vi "Handle Ctl[] Settings.vi"(7 "Write Ctl? (F:Read)":bool, 8 "error in (no error)":errorcluster, 10 "Controls[]":refnum<vi>[](array[refnum]), 11 "Save Restore Settings in":refnum<class "Save Restore Settings.lvclass">) -> (0 "error out":errorcluster, 3 "Save Restore Settings out":refnum<class "Save Restore Settings.lvclass">)   [LabVIEW 2020, in "Save Restore Settings.lvclass"]
uses:
  <userlib>/_MGI/Application Control/MGI Save Restore Settings/Save Restore Settings.lvclass
  <userlib>/_MGI/Application Control/MGI Save Restore Settings/Control Info.ctl
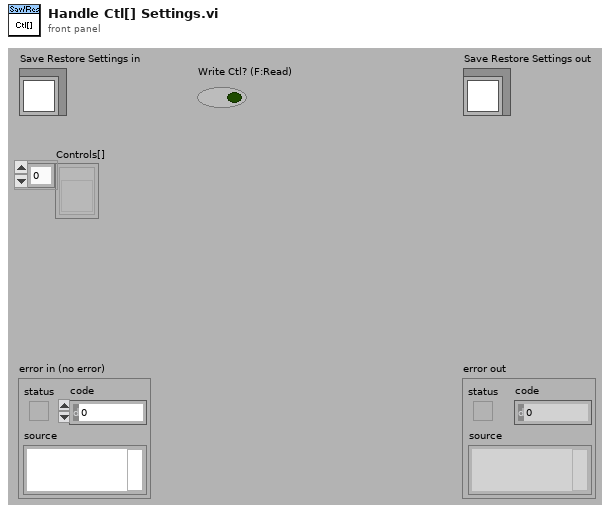
[diagram p1: front panel]
types:
  T1 = typedef "Save Restore Settings.lvclass/Control Info.ctl" = cluster{"Ref":refnum<vi>, "Tag":string}
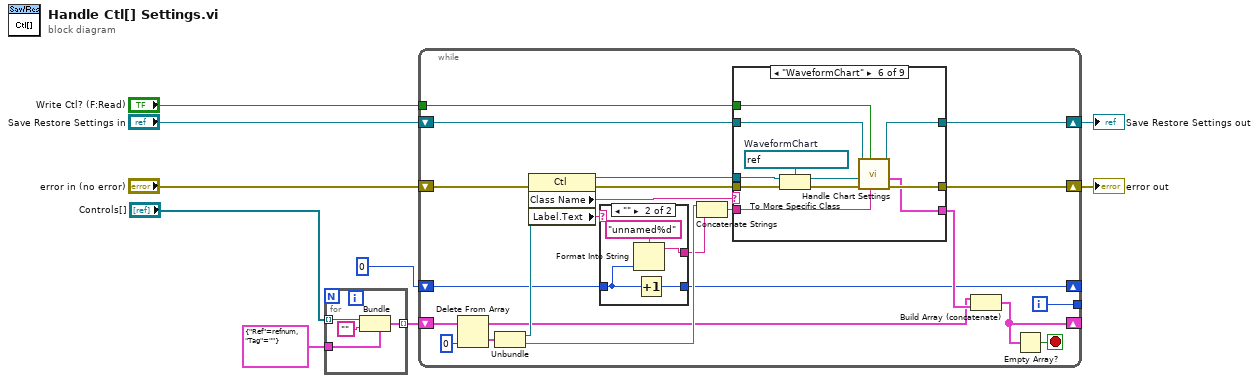
[diagram p0: block diagram]
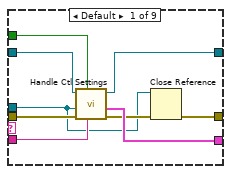
[diagram p3: hidden frame]
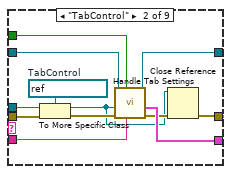
[diagram p4: hidden frame]
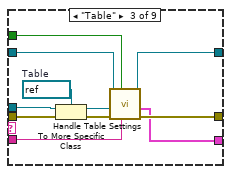
[diagram p5: hidden frame]
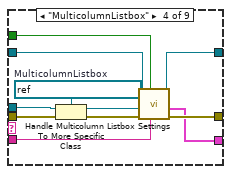
[diagram p6: hidden frame]
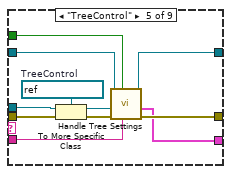
[diagram p7: hidden frame]
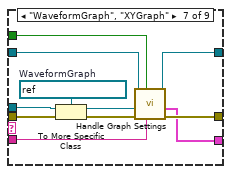
[diagram p8: hidden frame]
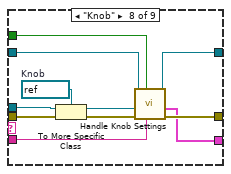
[diagram p9: hidden frame]
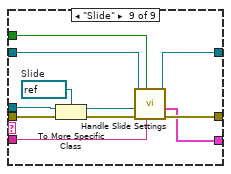
[diagram p10: hidden frame]
diagram:
  n1 = for {
    tunnel: "Controls[]" -> [w13] mode=indexing
    tunnel: [w12] -> w9 mode=indexing
    tunnel: T1 {"Ref"=refnum, "Tag"=""} ("Save Restore Settings.lvclass:Control Info") -> [w10]
    n2 = Bundle(cluster=w10, "Ref"=w13, "Tag"="") -> (w12:T1)
  }
  n3 = while {
    shift-right: [w23] -> _
    shift-left: w9 -> [w36]
    shift-right: [w28] -> w6
    shift-left: "error in (no error)" -> [w29]
    shift-right: [w25] -> w5
    shift-left: "Save Restore Settings in" -> [w26]
    shift-right: [w16] -> _
    shift-left: 0 -> [w18]
    tunnel: [w15] -> _
    tunnel: "Write Ctl? (F:Read)" -> [w14]
    i -> [w15]
    stop <- w27 stop-if-true
    n4 = Delete From Array(array=w36, index=0) -> (deleted portion=w35:T1, array with subset deleted=w20:T1[])  [unwired: 1 in]
    n5 = Unbundle(w35) -> ("Ref"=w22:refnum<vi>, "Tag"=w21:string)
    n6 = property class="Ctl"(reference=w22, error in=w29) -> (reference out=w33:refnum<vi>, error out=w34:errorcluster, "Class Name"=w32:string, "Label.Text"=w19:string)
    n7 = case shown="\"\"" w19 {
      selector: w19 -> [w38 _]
      tunnel: w18 -> [w37 w41]
      tunnel: [w38 w40] -> w17
      tunnel: [w37 w42] -> w16
      frame Default {
      }
      frame "" {
        n8 = Format Into String(format string="unnamed%d", w41) -> (resulting string=w40:string)  [unwired: 2 in, 1 out]
        n9 = Increment(x=w41) -> (x+1=w42:i32)
      }
    }
    n10 = Concatenate Strings(w21, w17) -> (w31:string)
    n11 = case shown="\"WaveformChart\"" w32 {
      tunnel: w34 -> [w51 w63 w73 w84 w95 w106 w117 w128 w139]
      tunnel: w31 -> [w50 w55 w69 w76 w87 w98 w109 w120 w131]
      tunnel: w33 -> [w44 w62 w72 w83 w94 w105 w116 w127 w138]
      tunnel: [w45 w60 w66 w78 w89 w100 w111 w122 w133] -> w28
      tunnel: w26 -> [w49 w59 w68 w81 w92 w103 w114 w125 w136]
      tunnel: [w48 w54 w67 w80 w91 w102 w113 w124 w135] -> w25
      tunnel: [w47 w57 w65 w77 w88 w99 w110 w121 w132] -> w24
      tunnel: w14 -> [w43 w52 w64 w75 w86 w97 w108 w119 w130]
      frame Default {
        n12 = call-dynamic "Handle Ctl Settings.vi"("Control Setting Tag"=w50, "Write? (F:Read)"=w43, "error in (no error)"=w51, "Control"=w44, "Save Restore Settings in"=w49) -> ("error out"=w46:errorcluster, "Sub Controls"=w47:T1[], "Save Restore Settings out"=w48:refnum<class "Save Restore Settings.lvclass">)  [unwired: 4 in]
        n13 = Close Reference(reference=w44, error in (no error)=w46) -> (error out=w45:errorcluster)
      }
      frame "TabControl" {
        w61 = refnum<vi> refnum  # TabControl
        n14 = To More Specific Class(target class=w61, reference=w62, error in=w63) -> (specific class reference=w53:refnum<vi>, error out=w58:errorcluster)
        n15 = call-dynamic "Handle Tab Settings.vi"("Tab Setting Name in"=w55, "Write? (F:Read)"=w52, "error in (no error)"=w58, "Tab"=w53, "Save Restore Settings in"=w59) -> ("error out"=w56:errorcluster, "Sub Controls"=w57:T1[], "Save Restore Settings out"=w54:refnum<class "Save Restore Settings.lvclass">)  [unwired: 4 in]
        n16 = Close Reference(reference=w53, error in (no error)=w56) -> (error out=w60:errorcluster)
      }
      frame "Table" {
        w74 = refnum<vi> refnum  # Table
        n17 = To More Specific Class(target class=w74, reference=w72, error in=w73) -> (specific class reference=w71:refnum<vi>, error out=w70:errorcluster)
        n18 = call-dynamic "Handle Table Settings.vi"("Table Setting Name in"=w69, "Write? (F:Read)"=w64, "error in (no error)"=w70, "Table Ref"=w71, "Save Restore Settings in"=w68) -> ("error out"=w66:errorcluster, "Sub Controls"=w65:T1[], "Save Restore Settings out"=w67:refnum<class "Save Restore Settings.lvclass">)  [unwired: 4 in]
      }
      frame "MulticolumnListbox" {
        w85 = refnum<vi> refnum  # MulticolumnListbox
        n19 = To More Specific Class(target class=w85, reference=w83, error in=w84) -> (specific class reference=w82:refnum<vi>, error out=w79:errorcluster)
        n20 = call-dynamic "Handle Multicolumn Listbox Settings.vi"("Table Setting Name in"=w76, "Write? (F:Read)"=w75, "error in (no error)"=w79, "Table Ref"=w82, "Save Restore Settings in"=w81) -> ("error out"=w78:errorcluster, "Sub Controls"=w77:T1[], "Save Restore Settings out"=w80:refnum<class "Save Restore Settings.lvclass">)  [unwired: 4 in]
      }
      frame "TreeControl" {
        w96 = refnum<vi> refnum  # TreeControl
        n21 = To More Specific Class(target class=w96, reference=w94, error in=w95) -> (specific class reference=w93:refnum<vi>, error out=w90:errorcluster)
        n22 = call-dynamic "Handle Tree Settings.vi"("Table Setting Name in"=w87, "Write? (F:Read)"=w86, "error in (no error)"=w90, "Table Ref"=w93, "Save Restore Settings in"=w92) -> ("error out"=w89:errorcluster, "Sub Controls"=w88:T1[], "Save Restore Settings out"=w91:refnum<class "Save Restore Settings.lvclass">)  [unwired: 4 in]
      }
      frame "WaveformChart" {
        w107 = refnum<vi> refnum  # WaveformChart
        n23 = To More Specific Class(target class=w107, reference=w105, error in=w106) -> (specific class reference=w104:refnum<vi>, error out=w101:errorcluster)
        n24 = call-dynamic "Handle Chart Settings.vi"("Table Setting Name in"=w98, "Write Ctl? (F:Read)"=w97, "error in (no error)"=w101, "Table Ref"=w104, "Save Restore Settings in"=w103) -> ("error out"=w100:errorcluster, "Sub Controls"=w99:T1[], "Save Restore Settings out"=w102:refnum<class "Save Restore Settings.lvclass">)  [unwired: 4 in]
      }
      frame "WaveformGraph", "XYGraph" {
        w118 = refnum<vi> refnum  # WaveformGraph
        n25 = To More Specific Class(target class=w118, reference=w116, error in=w117) -> (specific class reference=w115:refnum<vi>, error out=w112:errorcluster)
        n26 = call-dynamic "Handle Graph Settings.vi"("Table Setting Name in"=w109, "Write Ctl? (F:Read)"=w108, "error in (no error)"=w112, "Table Ref"=w115, "Save Restore Settings in"=w114) -> ("error out"=w111:errorcluster, "Sub Controls"=w110:T1[], "Save Restore Settings out"=w113:refnum<class "Save Restore Settings.lvclass">)  [unwired: 4 in]
      }
      frame "Knob" {
        w129 = refnum<vi> refnum  # Knob
        n27 = To More Specific Class(target class=w129, reference=w127, error in=w128) -> (specific class reference=w126:refnum<vi>, error out=w123:errorcluster)
        n28 = call-dynamic "Handle Knob Settings.vi"("Table Setting Name in"=w120, "Write? (F:Read)"=w119, "error in (no error)"=w123, "Knob"=w126, "Save Restore Settings in"=w125) -> ("error out"=w122:errorcluster, "Sub Controls"=w121:T1[], "Save Restore Settings out"=w124:refnum<class "Save Restore Settings.lvclass">)  [unwired: 4 in]
      }
      frame "Slide" {
        w140 = refnum<vi> refnum  # Slide
        n29 = To More Specific Class(target class=w140, reference=w138, error in=w139) -> (specific class reference=w137:refnum<vi>, error out=w134:errorcluster)
        n30 = call-dynamic "Handle Slide Settings.vi"("Table Setting Name in"=w131, "Write? (F:Read)"=w130, "error in (no error)"=w134, "Knob"=w137, "Save Restore Settings in"=w136) -> ("error out"=w133:errorcluster, "Sub Controls"=w132:T1[], "Save Restore Settings out"=w135:refnum<class "Save Restore Settings.lvclass">)  [unwired: 4 in]
      }
    }
    n31 = Build Array (concatenate)(w20, w24) -> (w23:T1[])
    n32 = Empty Array?(array=w23) -> (empty?=w27:bool)
  }
  "error out" <- w6
  "Save Restore Settings out" <- w5
